vi "2 SailControlFunction.vi"() -> (2 "Sail Position":T1)   [LabVIEW 2011]
doc: "Sets the desired sail position based on the apparent wind direction.\nDesired sail position is same from 0-4 degrees, 5-9 degrees, and so on and so forth.\nValues come from a lookup table, which hopefully will make it easier to change if experimentation calls for different set values."
uses:
  2 Typedefs/sail setpt.ctl
  2 Typedefs/Which Boat.ctl
  2 Typedefs/apparent wind direction.ctl
  2 Globals/2 Global.vi
panel:
  out "Apparent Wind Dir":T1
  in  "Sail Setpoint Lookup Table Small RC":dbl[][](array[numeric])=[[0.0, 0.0, 0.0, 0.0, 0.0, 0.0, 0.0, 0.0, 0.0, 0.0, 0.055, 0.111, 0.166, 0.222, 0.277, 0.333, 0.388, 0.444, 0.5, 0.5278, 0.5556, 0.5833, 0.6111, 0.6389, 0.6667, 0.6944, 0.7222, 0.75, 0.7778, 0.8056, 0.8333, 0.8611, 0.8889, 0.9167, 0.9444, 0.9722, 1.0], [1.0, 0.9722, 0.9444, 0.9167, 0.8889, 0.8611, 0.8333, 0.8056, 0.7778, 0.75, 0.7222, 0.6944, 0.6667, 0.6389, 0.6111, 0.5833, 0.5556, 0.5278, 0.5, 0.4444, 0.3889, 0.3333, 0.2778, 0.2222, 0.1667, 0.1111, 0.0556, 0.0, 0.0, 0.0, 0.0, 0.0, 0.0, 0.0, 0.0, 0.0, 0.0]]
  in  "Sail Setpoint Lookup Table Competition Boat":dbl[][](array[numeric])=[[0.0, 0.0, 0.0, 0.0, 0.0, 0.0, 0.0, 0.0, 0.0, 0.0, 0.055, 0.111, 0.166, 0.222, 0.277, 0.333, 0.388, 0.444, 0.5, 0.5278, 0.5556, 0.5833, 0.6111, 0.6389, 0.6667, 0.6944, 0.7222, 0.75, 0.7778, 0.8056, 0.8333, 0.8611, 0.8889, 0.9167, 0.9444, 0.9722, 1.0], [1.0, 0.9722, 0.9444, 0.9167, 0.8889, 0.8611, 0.8333, 0.8056, 0.7778, 0.75, 0.7222, 0.6944, 0.6667, 0.6389, 0.6111, 0.5833, 0.5556, 0.5278, 0.5, 0.4444, 0.3889, 0.3333, 0.2778, 0.2222, 0.1667, 0.1111, 0.0556, 0.0, 0.0, 0.0, 0.0, 0.0, 0.0, 0.0, 0.0, 0.0, 0.0]]
  out "Which Boat Am I?":T2
  # "First row is 0-180\nSecond row is 180-360, and in theory should be equal to the first one. Experiments must be run to determine if this is true."
  # "Currently 0 from 0-45, straight line 50 - 90 (.5), straight line 95 - 180 (1)"
  # "90"
  # "135"
  # "180"
  # "225"
  # "270"
  # "315"
  # "360"
  # "90"
  # "180"
  # "135"
  # "270"
  # "225"
  # "315"
  # "360"
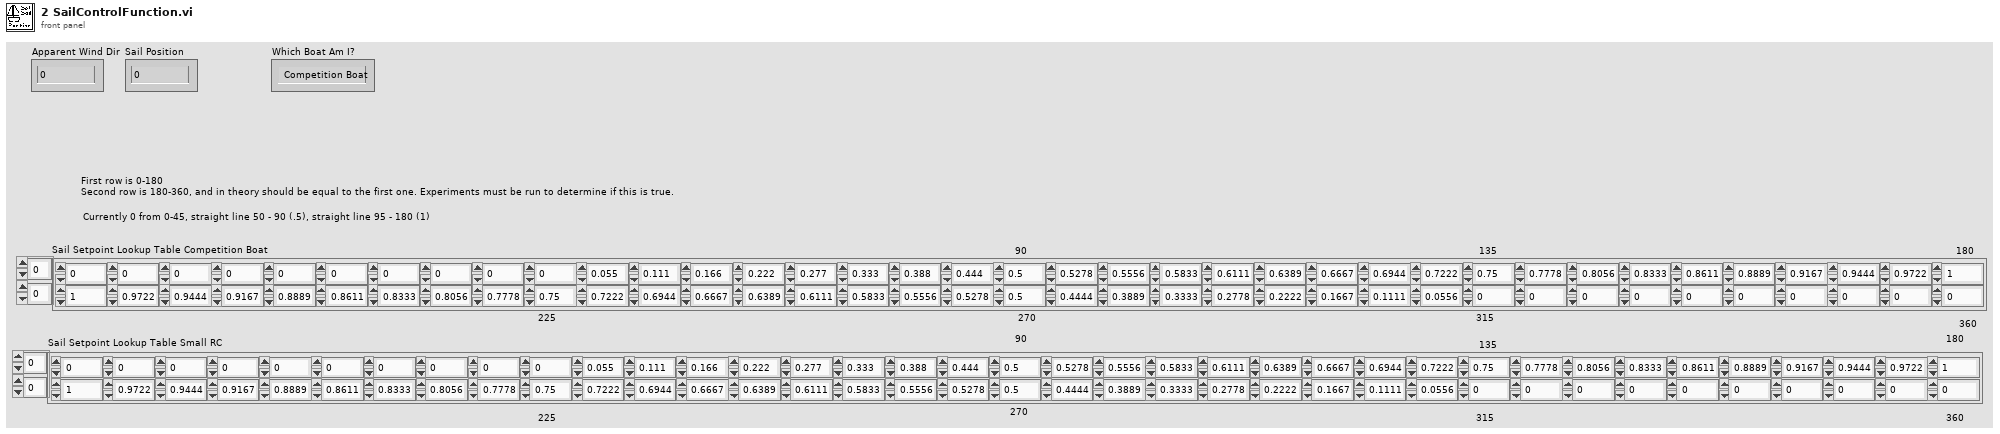
[diagram p1: front panel]
types:
  T1 = typedef "sail setpt.ctl" = dbl
  T2 = typedef "Which Boat.ctl" = enum16{"Competition Boat", "Small RC", "Simulation"}
  T3 = typedef "apparent wind direction.ctl" = dbl
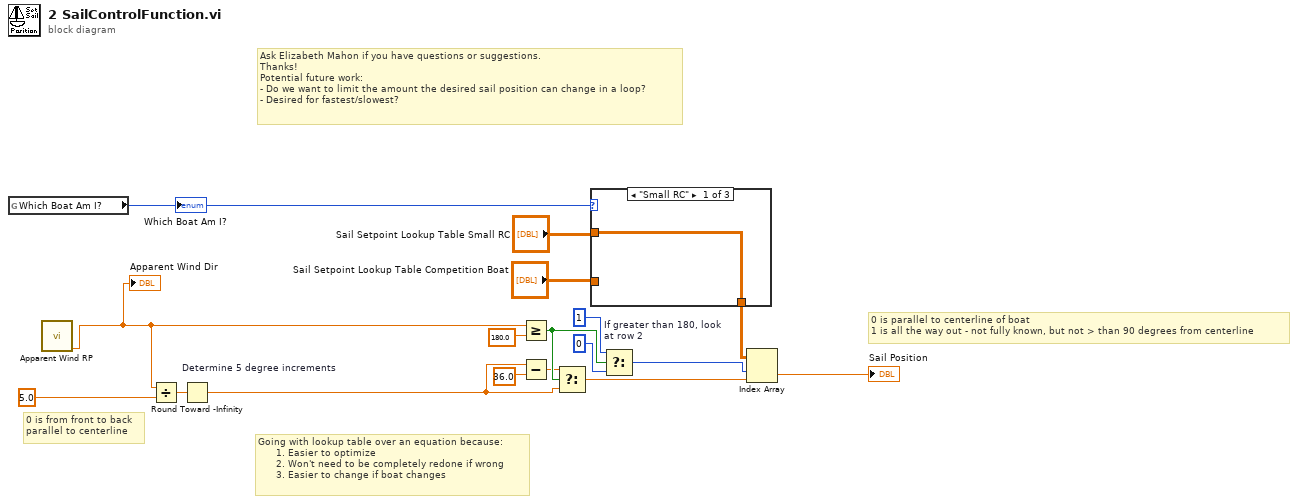
[diagram p0: block diagram]
diagram:
  # "0 is from front to back\nparallel to centerline"
  # "Ask Elizabeth Mahon if you have questions or suggestions.\nThanks!\nPotential future work:\n- Do we want to limit the amount the desired sail position can change in a loop?\n- Desired for fastest/slowest?"
  # "0 is parallel to centerline of boat\n1 is all the way out - not fully known, but not > than 90 degrees from centerline"
  # "Going with lookup table over an equation because:\n      1. Easier to optimize\n      2. Won't need to be completely redone if wrong\n      3. Easier to change if boat changes"
  n1 = global read "2 Global.vi" "Which Boat Am I?"() -> (w2:T2)
  "Which Boat Am I?" <- w2
  n2 = call "Apparent Wind RP.vi"() -> ("Apparent Wind Direction RP"=w1:dbl)  [unwired: 8 in, 3 out]
  "Apparent Wind Dir" <- w1
  n3 = Divide(x=w1, y=T3 5.0) -> (x/y=w15:T3)
  n4 = Round Toward -Infinity "Determine 5 degree increments"(1:w15) -> (0:w6:T3)
  n5 = Greater Or Equal?(x=w1, y=T3 180.0) -> (x >= y?=w9:bool)
  n6 = Subtract(x=w6, y=T3 36.0) -> (x-y=w7:T3)
  n7 = Select(t=w7, s=w9, f=w6) -> (s? t:f=w5:T3)
  n8 = case shown="\"Small RC\"" w2 {
    tunnel: [w18 w19 w20] -> w10
    tunnel: "Sail Setpoint Lookup Table Competition Boat" -> [_ w19 w20]
    tunnel: "Sail Setpoint Lookup Table Small RC" -> [w18 _ _]
    frame "Small RC" {
    }
    frame "Simulation" {
    }
    frame "Competition Boat" {
    }
  }
  n9 = Select "If greater than 180, look\nat row 2"(t=1, s=w9, f=0) -> (s? t:f=w11:i32)
  n10 = Index Array(array=w10, index (row)=w11, index (col)=w5) -> (element=→"Sail Position":dbl)
